vi "test_PV_Wf.vi"() -> ()   [LabVIEW 2013]
panel:
  out "size(s)":i32
  in  "stop":bool
  out "data":dbl[](array[numeric])
  out "SR Fill Pattern":dbl[](graph)
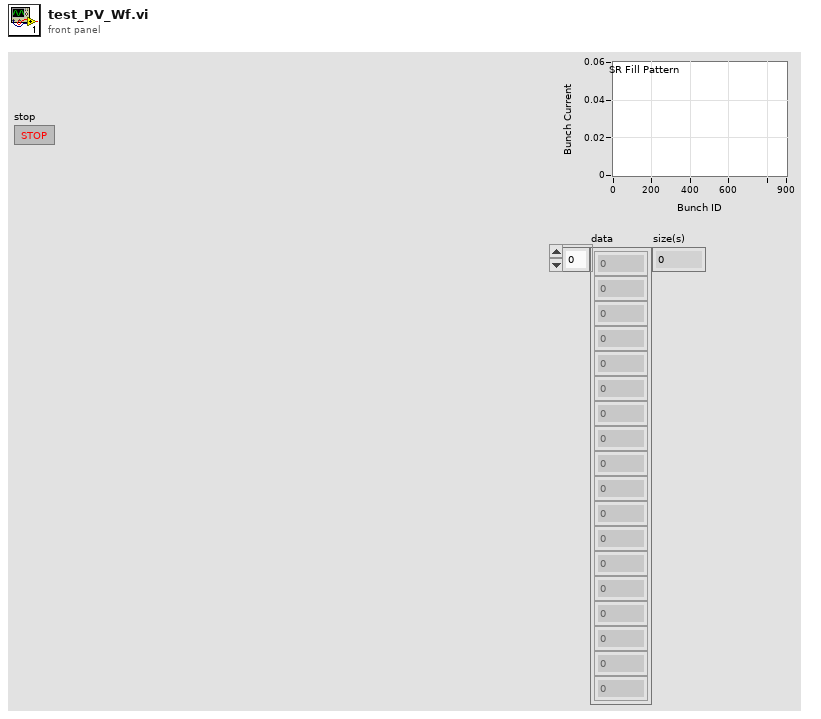
[diagram p1: front panel]
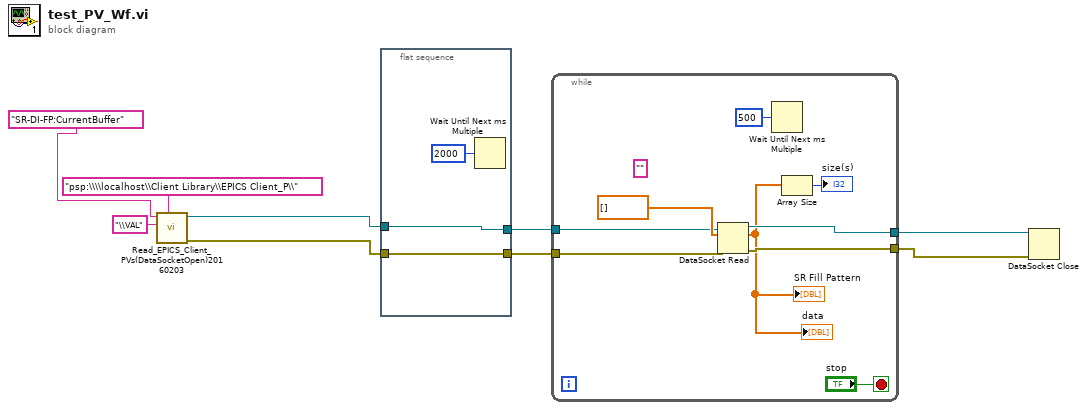
[diagram p0: block diagram]
diagram:
  n1 = call "Read_EPICS_Client_PVs(DataSocketOpen)20160203.vi"("LLB"="psp:\\\\localhost\\Client Library\\EPICS Client_P\\", "field"="\\VAL", "PV name"="SR-DI-FP:CurrentBuffer") -> ("error out"=w1:errorcluster, "connection id"=w3:refnum<k13>)  [unwired: 7 in]
  n2 = flat-sequence {
    tunnel: [w12] -> w4
    tunnel: w3 -> [w12]
    tunnel: [w11] -> w2
    tunnel: w1 -> [w11]
    frame #0 {
      n3 = Wait Until Next ms Multiple(millisecond multiple=u32 2000) -> ()  [unwired: 1 out]
    }
  }
  n4 = while {
    tunnel: w4 -> [w20]
    tunnel: [w19] -> w7
    tunnel: [w18] -> w6
    tunnel: w2 -> [w17]
    stop <- "stop" stop-if-true
    (unwired) ""
    n5 = DataSocket Read(8:w17, 10:dbl[] [], 11:w20) -> (0:w18:errorcluster, 2:w14:dbl[], 3:w19:refnum<k13>)  [unwired: 2 in, 4 out]
    "SR Fill Pattern" <- w14
    "data" <- w14
    n6 = Wait Until Next ms Multiple(millisecond multiple=u32 500) -> ()  [unwired: 1 out]
    n7 = Array Size(array=w14) -> (size(s)=→"size(s)":i32)
  }
  n8 = DataSocket Close(8:w6, 11:w7) -> ()  [unwired: 1 in, 2 out]
